vi "Assert Stop.vi"(8 "error in (no error)":errorcluster, 10 "stop (F)":bool, 11 "Stop Pointer in":refnum<class "Stop Pointer.lvclass">) -> (0 "error out":errorcluster, 2 "stop?":bool, 3 "Stop Pointer out":refnum<class "Stop Pointer.lvclass">)   [LabVIEW 2017, in "Memory Manager.lvlib" / "Stop Pointer.lvclass"]
doc: "Writes the value of <b>stop</b> to the provided <b>Stop Pointer</b> only if the value is TRUE. The current value of the stop pointer is then returned."
uses:
  Stop Pointer.lvclass
  C:/Git/LabVIEW-Memory/Source/Classes/Pointer/Pointer.lvclass
  Read Bool.vi
  Write Bool.vi
  Pointer.lvclass
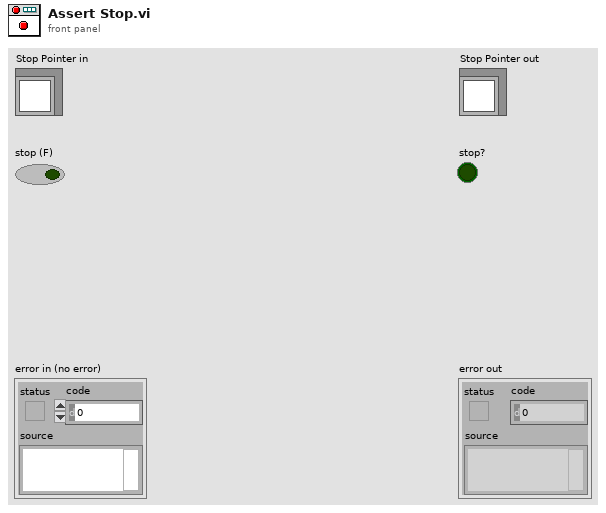
[diagram p1: front panel]
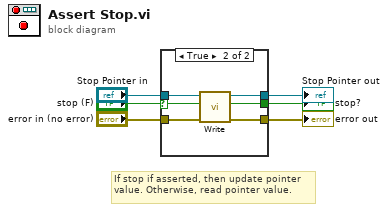
[diagram p0: block diagram]
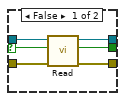
[diagram p2: hidden frame]
diagram:
  # "If stop if asserted, then update pointer value. Otherwise, read pointer value."
  n1 = case shown="True" "stop (F)" {
    selector: "stop (F)" -> [w7 w13]
    tunnel: "Stop Pointer in" -> [w12 w18]
    tunnel: "error in (no error)" -> [w11 w17]
    tunnel: [w10 w16] -> w4
    tunnel: [w9 w15] -> w3
    tunnel: [w8 w14] -> w2
    frame False {
      n2 = call-poly "Read.vi"("error in (no error)"=w11, "value in"=w7, "Pointer in"=w12) -> ("error out"=w9:errorcluster, "value out"=w8:bool, "Pointer out"=w10:refnum<class "Stop Pointer.lvclass">)  [unwired: 5 in, 1 out]
    }
    frame True {
      n3 = call-poly "Write.vi"("error in (no error)"=w17, "value"=w13, "Pointer in"=w18) -> ("error out"=w15:errorcluster, "value"=w14:bool, "Pointer out"=w16:refnum<class "Stop Pointer.lvclass">)  [unwired: 5 in, 1 out]
    }
  }
  "error out" <- w3
  "Stop Pointer out" <- w4
  "stop?" <- w2
